vi "Write Meta Data (TCP Clst).vi"(6 "options":T3={"ignore timeout error"=TRUE, "timeout ms (1000)"=1000}, 7 "meta data":T2[](array[typedef]), 8 "error in":errorcluster, 11 "connection info in":T1) -> (0 "error out":errorcluster, 3 "connection info out":T1)   [LabVIEW 2013, in "NI STM.lvlib"]
doc: "Use this VI to transmit the meta data cluster to a remote computer. Sending the meta data to another computer helps maintainability since the data resides only on one side and it is shared to other computers at run time."
uses:
  NI STM.lvlib
  TCP Connection Info.ctl
  SubVIs/MetaDataElement.ctl
  TCP Write Options.ctl
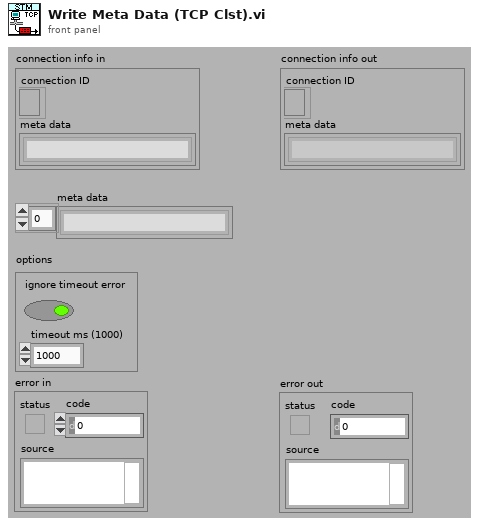
[diagram p1: front panel]
types:
  T1 = typedef "NI STM.lvlib/TCP Connection Info.ctl" = cluster{"connection ID":refnum<k5>, "meta data":T2[]}
  T2 = typedef "NI STM.lvlib/MetaDataElement.ctl" = string
  T3 = typedef "NI STM.lvlib/TCP Write Options.ctl" = cluster{"ignore timeout error":bool, "timeout ms (1000)":i32}
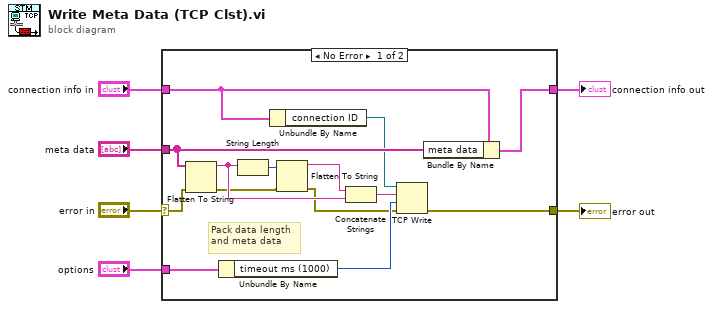
[diagram p0: block diagram]
diagram:
  n1 = case shown="No Error" "error in" {
    selector: "error in" -> [w11 w22]
    tunnel: [w13 w21] -> w6
    tunnel: "connection info in" -> [w8 w21]
    tunnel: "meta data" -> [w12 _]
    tunnel: [w20 w22] -> w4
    tunnel: "options" -> [w15 _]
    frame No Error {
      # "Pack data length\nand meta data"
      n2 = Flatten To String(anything=w12, error in (no error)=w11) -> (data string=w16:string, error out=w10:errorcluster)  [unwired: 3 out]
      n3 = Unbundle By Name(w15) -> ("timeout ms (1000)"=w14:i32)
      n4 = String Length(string=w16) -> (length=w19:i32)
      n5 = Unbundle By Name(w8) -> ("connection ID"=w7:refnum<k5>)
      n6 = Flatten To String(anything=w19, error in (no error)=w10) -> (data string=w18:string, error out=w9:errorcluster)  [unwired: 3 out]
      n7 = Concatenate Strings(w18, w16) -> (w17:string)
      n8 = TCP Write(connection ID=w7, data in=w17, error in (no error)=w9, 9:w14) -> (error out=w20:errorcluster)  [unwired: 2 out]
      n9 = Bundle By Name(cluster=w8, "meta data"=w12) -> (w13:T1)
    }
    frame Error {
    }
  }
  "connection info out" <- w6
  "error out" <- w4
